vi "TDTSyn-Get Waves.vi"(0 "State In":T1, 7 "codes":string, 9 "last":bool, 11 "error in (no error)":errorcluster) -> (4 "State Out":T1, 8 "Waves":dbl[][](array[numeric]), 15 "error out":errorcluster)   [LabVIEW 2020]
uses:
  TDTSyn-State.ctl
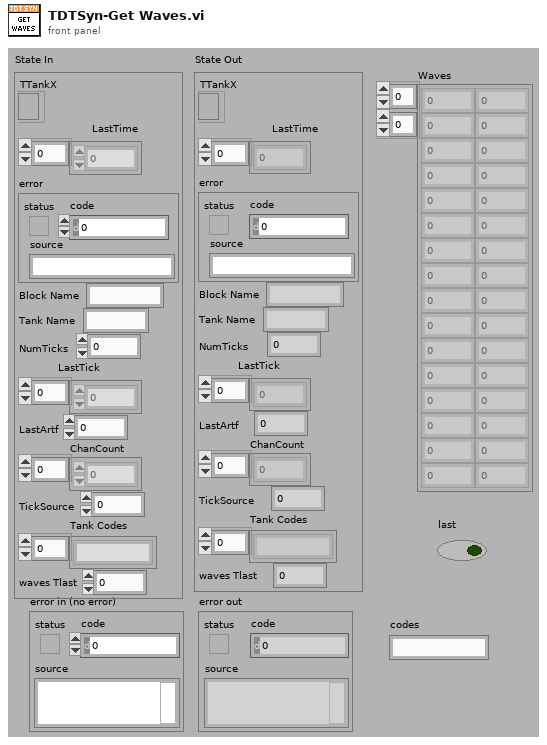
[diagram p1: front panel]
types:
  T1 = typedef "TDTSyn-State.ctl" = cluster{"TTankX":refnum<k7>, "LastTime":dbl[], "error":errorcluster, "Block Name":string, "Tank Name":string, "NumTicks":i32, "LastTick":dbl[], "LastArtf":dbl, "ChanCount":i32[], "TickSource":i32, "Tank Codes":string[], "waves Tlast":dbl}
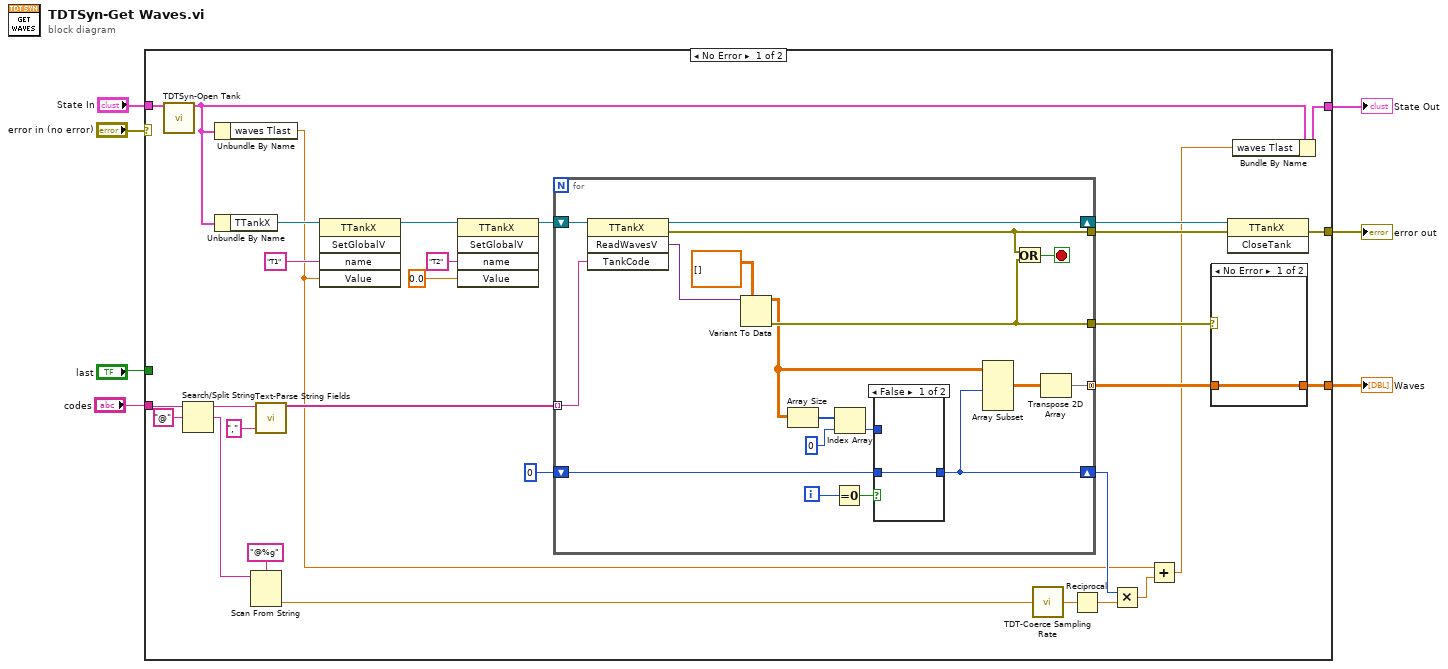
[diagram p0: block diagram]
diagram:
  n1 = case shown="No Error" "error in (no error)" {
    selector: "error in (no error)" -> [_ w60]
    tunnel: [w36 w60] -> w6
    tunnel: "State In" -> [w37 w59]
    tunnel: [w23 w59] -> w4
    tunnel: "codes" -> [w13 _]
    tunnel: [w30 _] -> w2
    tunnel: "last" -> [_ _]
    frame No Error {
      n2 = call "TDTSyn-Open Tank.vi"("State In"=w37) -> ("State Out"=w24:T1)  [unwired: 13 in, 1 out]
      n3 = Search/Split String(string=w13, search string/char (-)="@") -> (substring before match=w12:string, match + rest of string=w9:string)  [unwired: 1 in, 1 out]
      n4 = Unbundle By Name(w24) -> ("waves Tlast"=w14:dbl)
      n5 = Unbundle By Name(w24) -> ("TTankX"=w29:refnum<k7>)
      n6 = Scan From String(format string="@%g", input string=w9) -> (output 1=w8:dbl)  [unwired: 3 in, 3 out]
      n7 = call "Text-Parse String Fields.vi"("String"=w12, "Separator"=",") -> ("Fields"=w35:string[])  [unwired: 8 in, 5 out]
      n8 = invoke class="TTankX" method="SetGlobalV"(reference=w29, "name"="T1", "Value"=w14) -> (reference out=w25:refnum<k7>)  [unwired: 2 in, 4 out]
      n9 = invoke class="TTankX" method="SetGlobalV"(reference=w25, "name"="T2", "Value"=0.0) -> (reference out=w26:refnum<k7>)  [unwired: 2 in, 4 out]
      n10 = for {
        tunnel: w35 -> [w54] mode=indexing
        shift-right: [w53] -> w33
        shift-left: w26 -> [w55]
        tunnel: [w50] -> w32
        tunnel: [w49] -> w31
        shift-right: [w42] -> w17
        shift-left: 0 -> [w44]
        tunnel: [w38] -> w16 mode=concatenating
        i -> [w46]
        stop <- w48 stop-if-true
        n11 = invoke class="TTankX" method="ReadWavesV"(reference=w55, "TankCode"=w54) -> (reference out=w53:refnum<k7>, error out=w50:errorcluster, "ReadWavesV"=w51:variant)  [unwired: 2 in, 1 out]
        n12 = Variant To Data(type=sgl[][] [], Variant=w51) -> (data=w47:sgl[][], error out=w49:errorcluster)  [unwired: 1 in]
        n13 = Array Size(array=w47) -> (size(s)=w45:i32[])
        n14 = Equal To 0?(x=w46) -> (x = 0?=w43:bool)
        n15 = Index Array(array=w45, index=0) -> (element=w40:i32)
        n16 = case shown="False" w43 {
          tunnel: w40 -> [_ w57]
          tunnel: w44 -> [w56 _]
          tunnel: [w56 w57] -> w42
          frame False {
          }
          frame True {
          }
        }
        n17 = Array Subset(array=w47, length (row)=w42) -> (w41:sgl[][])  [unwired: 3 in]
        n18 = Or(x=w50, y=w49) -> (x .or. y?=w48:bool)
        n19 = Transpose 2D Array(2D array=w41) -> (transposed array=w38:sgl[][])
      }
      n20 = call "TDT-Coerce Sampling Rate.vi"("Fs (Hz)"=w8) -> ("Coerced"=w21:dbl)
      n21 = Reciprocal(x=w21) -> (1/x=w20:dbl)
      n22 = Multiply(x=w17, y=w20) -> (x*y=w19:dbl)
      n23 = Add(x=w14, y=w19) -> (x+y=w15:dbl)
      n24 = case shown="No Error" w31 {
        tunnel: w16 -> [w58 _]
        tunnel: [w58 _] -> w30
        frame No Error {
        }
        frame Error {
        }
      }
      n25 = invoke class="TTankX" method="CloseTank"(reference=w33, error in=w32) -> (error out=w36:errorcluster)  [unwired: 1 in, 2 out]
      n26 = Bundle By Name(cluster=w24, "waves Tlast"=w15) -> (w23:T1)
    }
    frame Error {
    }
  }
  "error out" <- w6
  "State Out" <- w4
  "Waves" <- w2
